vi "AssertSubtexts.vi"(7 "Expected":string[](array[string]), 8 "error in":errorcluster, 10 "offset":i32, 11 "string":string) -> (0 "error out":errorcluster, 2 "offset out":i32, 3 "string copy":string, 5 "Which found":i32)   [LabVIEW 2020]
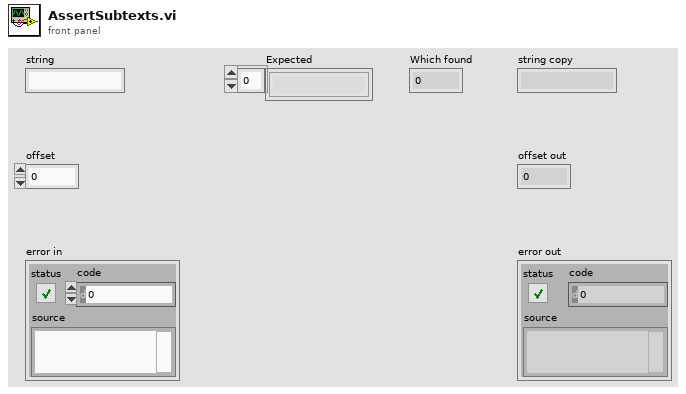
[diagram p1: front panel]
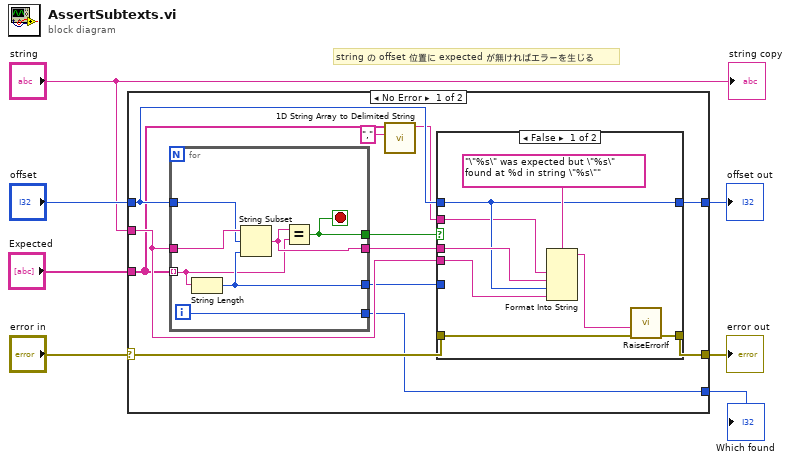
[diagram p0: block diagram]
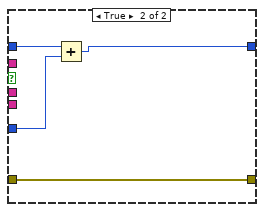
[diagram p2: hidden frame]
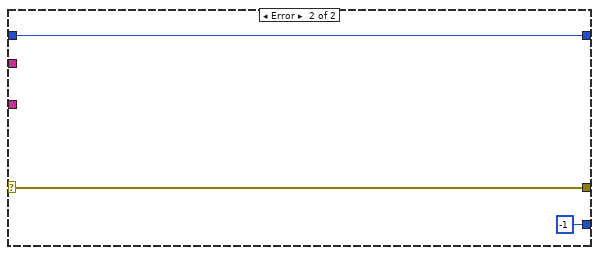
[diagram p3: hidden frame]
diagram:
  # "string の offset 位置に expected が無ければエラーを生じる"
  n1 = case shown="No Error" "error in" {
    selector: "error in" -> [w18 w41]
    tunnel: "offset" -> [w14 w40]
    tunnel: "string" -> [w16 _]
    tunnel: [w17 w41] -> w4
    tunnel: [w13 w40] -> w3
    tunnel: "Expected" -> [w12 _]
    tunnel: [w8 -1] -> w1
    frame No Error {
      n2 = for {
        tunnel: [w21] -> w19
        tunnel: [w24] -> w15
        tunnel: w14 -> [w23]
        tunnel: w12 -> [w22] mode=indexing
        tunnel: w16 -> [w26]
        tunnel: [w25] -> w9
        tunnel: [w20] -> w8
        i -> [w20]
        stop <- w21 stop-if-true
        n3 = String Length(string=w22) -> (length=w24:i32)
        n4 = String Subset(string=w26, offset (0)=w23, length (rest)=w24) -> (substring=w25:string)
        n5 = Equal?(x=w25, y=w22) -> (x = y?=w21:bool)
      }
      n6 = call <vilib>:"1D String Array to Delimited String.vi"("delimiter"=",", "string array"=w12) -> ("delimited string"=w10:string)  [unwired: 9 in]
      n7 = case shown="False" w19 {
        tunnel: w18 -> [w34 w38]
        tunnel: [w33 w38] -> w17
        tunnel: w16 -> [w30 _]
        tunnel: w9 -> [w31 _]
        tunnel: w14 -> [w29 w36]
        tunnel: w15 -> [_ w37]
        tunnel: [w29 w35] -> w13
        tunnel: w10 -> [w27 _]
        frame False {
          n8 = Format Into String(format string="\"%s\" was expected but \"%s\" found at %d in string \"%s\"", w27, w31, w29, w30) -> (resulting string=w28:string)  [unwired: 2 in, 1 out]
          n9 = call "RaiseErrorIf.vi"("error in (no error)"=w34, "error message"=w28) -> ("error out"=w33:errorcluster)  [unwired: 9 in]
        }
        frame True {
          n10 = Add(x=w36, y=w37) -> (x+y=w35:i32)
        }
      }
    }
    frame Error {
    }
  }
  "offset out" <- w3
  "error out" <- w4
  "Which found" <- w1
  "string copy" <- "string"
